vi "Set Center Frequency.vi"(8 "error in (no error)":errorcluster, 10 "Center Frequency":u32, 11 "DeviceRefnum":u64) -> (0 "error out":errorcluster, 2 "function return":i32, 3 "DeviceRefnum Out":u64)   [LabVIEW 2017]
doc: "Set the center frequency of the tuner."
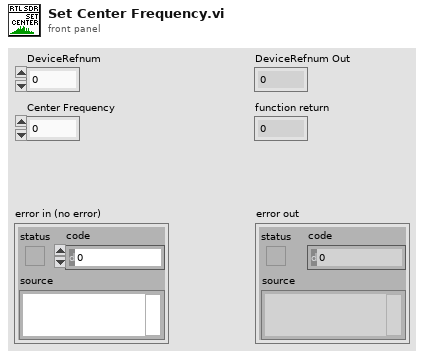
[diagram p1: front panel]
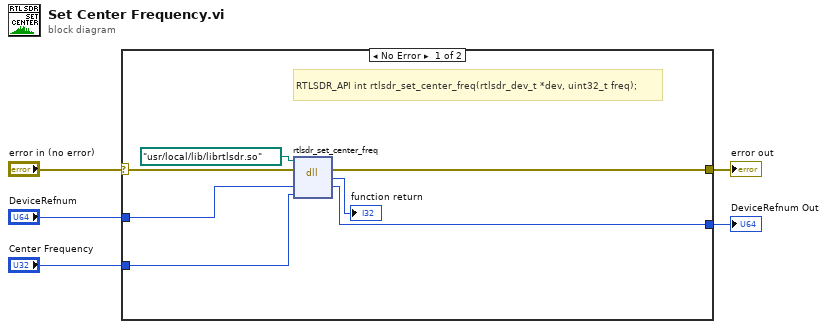
[diagram p0: block diagram]
diagram:
  n1 = case shown="No Error" "error in (no error)" {
    selector: "error in (no error)" -> [w7 w14]
    tunnel: "Center Frequency" -> [w11 _]
    tunnel: [w10 w14] -> w4
    tunnel: "DeviceRefnum" -> [w9 w13]
    tunnel: [w8 w13] -> w2
    frame No Error {
      # "RTLSDR_API int rtlsdr_set_center_freq(rtlsdr_dev_t *dev, uint32_t freq);"
      n2 = dll-call lib="C:/Program Files (x86)/National Instruments/LabVIEW 2016/user.lib/rtlsdr/rtlsdr.*" fn="rtlsdr_set_center_freq"(path in=path "/usr/local/lib/librtlsdr.so", error in=w7, "DeviceRefnum"=w9, "CenterFrequency"=w11) -> (error out=w10:errorcluster, "return type"=→"function return":i32, "DeviceRefnum"=w8:u64)  [unwired: 2 in, 1 out]
    }
    frame Error {
    }
  }
  "error out" <- w4
  "DeviceRefnum Out" <- w2
